vi "HEWH Create Header File.vi"(8 "Supply Voltage:":string, 9 "Test_Type:":string, 10 "HEWH Output Information":T1={"Scan Rate Adjust"=1000.0, "Draw Count"=0, "Test Patten Setup"={"Dispense Times"=[0.0, 3600.0, 7200.0, 10800.0, 14400.0, 18000.0], "Total Gallons Schedule"=[10.72, 10.72, 10.72, 10.72, 10.72, 10.72], "Flow Rate Schedule "=[3.0, 3.0, 3.0, 3.0, 3.0, 3.0], "Incoming Water Temperature"=[58.0, 58.0, 58.0, 58.0, 58.0, 58.0], "PreDraw Pattern"=[], "24 Hour PreDraw"=enum."Zero Pre-Draws", "Pre-Draw Until?"=[], "Purge Until Cutout"=FALSE, "Heating Flag"=FALSE}, "Condition Cluster Output"={"Condition #1"=FALSE, "Condition #2"=FALSE, "Special Last Draw (HU Test)"=FALSE, "RTD Out Temperature <="=0.0, "Condition #3"=FALSE, "Mean Tank Temperature <="=0.0, "Condition #4"=FALSE, "Decrease Outlet Temperature \nBy (RTD Out)"=0.0, "Condition #5"=FALSE, "Condition #6"=FALSE, "Time (Seconds)"=0.0, "Condition #7"=FALSE, "Condition #8"=FALSE, "Draw Until Condition"={"UE"=FALSE, "LE"=FALSE, "COMP"=FALSE, "FANS"=FALSE}, "Condition #9"=FALSE}, "HEWH Specific DAQ"={"HEWH Data"={"Voltage (Volts)"=-1.0, "Current (Amps)"=-1.0, "Power (Watts)"=-1.0, "WattHours (Wh)"=-1.0, "TC Tree (AVG)"=0.0, "Flow Rate (GPM)"=0.0, "Gallons (Gal)"=0.0, "RTD Out (Deg F)"=0.0, "TC Down"=0.0, "TC Tree Array"=[], "UE Event Lead"=0, "LE Event Lead"=0}, "Intellif Valve % Open"=0.0, "Power State"={"UE"=FALSE, "LE"=FALSE, "COMP"=FALSE, "FANS"=FALSE}, "Power Analyzer"=enum."APLUS", "Intellifaucet Configuration"=enum."DRK375,STATION3,1/2\"HOSE"}, "Test Output Data"={"PreDraw Data Table"=[], "Data Table"=[], "MW100 TC Headers"=[]}, "Calc and Calibration"={"RTD Max Min Array"=[], "Draw Statistics"=[], "Calibration Coefficients DBL"=[], "Min RTD Temp\nDuring Draw"=0.0, "Start Gallons"=0.0, "Starting Temp Decline Temp"=0.0, "Max RTD Temp\nDuring Draw"=0.0, "Draw Start Time"=0.0, "Delay Start Time"=0.0, "Current Purge Start Time"=0.0}, "Current Draw Time"=0.0} {"Test Patten Setup"."Incoming Water Temperature" format="%.2f"; "Test Patten Setup"."Flow Rate Schedule" format="%.2f"; "Test Patten Setup"."Total Gallons Schedule" format="%.2f"; "Test Patten Setup"."Dispense Times" format="%<%H:%M:%S>t"}) -> (3 "File Initialization Array":string[][](array[string]))   [LabVIEW 2016]
uses:
  Hybrid Water Heater/Type Definitions/HEWH Output Information.ctl
  Hybrid Water Heater/Type Definitions/HEWH Power Data.ctl
  Hybrid Water Heater/Type Definitions/HEWH Draw Pattern Setup.ctl
  Hybrid Water Heater/Type Definitions/HEWH Power Elements.ctl
  Hybrid Water Heater/Type Definitions/HEWH Termination Condition Cluster.ctl
  Hybrid Water Heater/Type Definitions/HEWH PreDraw.ctl
  Type Definitions/UTILITY Power Analyzer.ctl
  Hybrid Water Heater/Custom Instrument Control/Intellifaucet/Type Definitions/INTELLIFAUCET Tested Flowrate Scenarios.ctl
panel:
  # "Select Only One Condition"
  # "Just Draw Water!"
  # "Condition #1"
  # "Draw Until Any Heat Source"
  # "Condition #2"
  # "Start Dispense Pattern"
  # "Draw Until Specific Heat Source"
  # "Condition #3"
  # "Dispense PRAT Sequence"
  # "Not Working"
  # "Condition #4"
  # "Condition #5"
  # "Condition #6"
  # "Draw Pattern Setup"
  # "Pre-Draw Items"
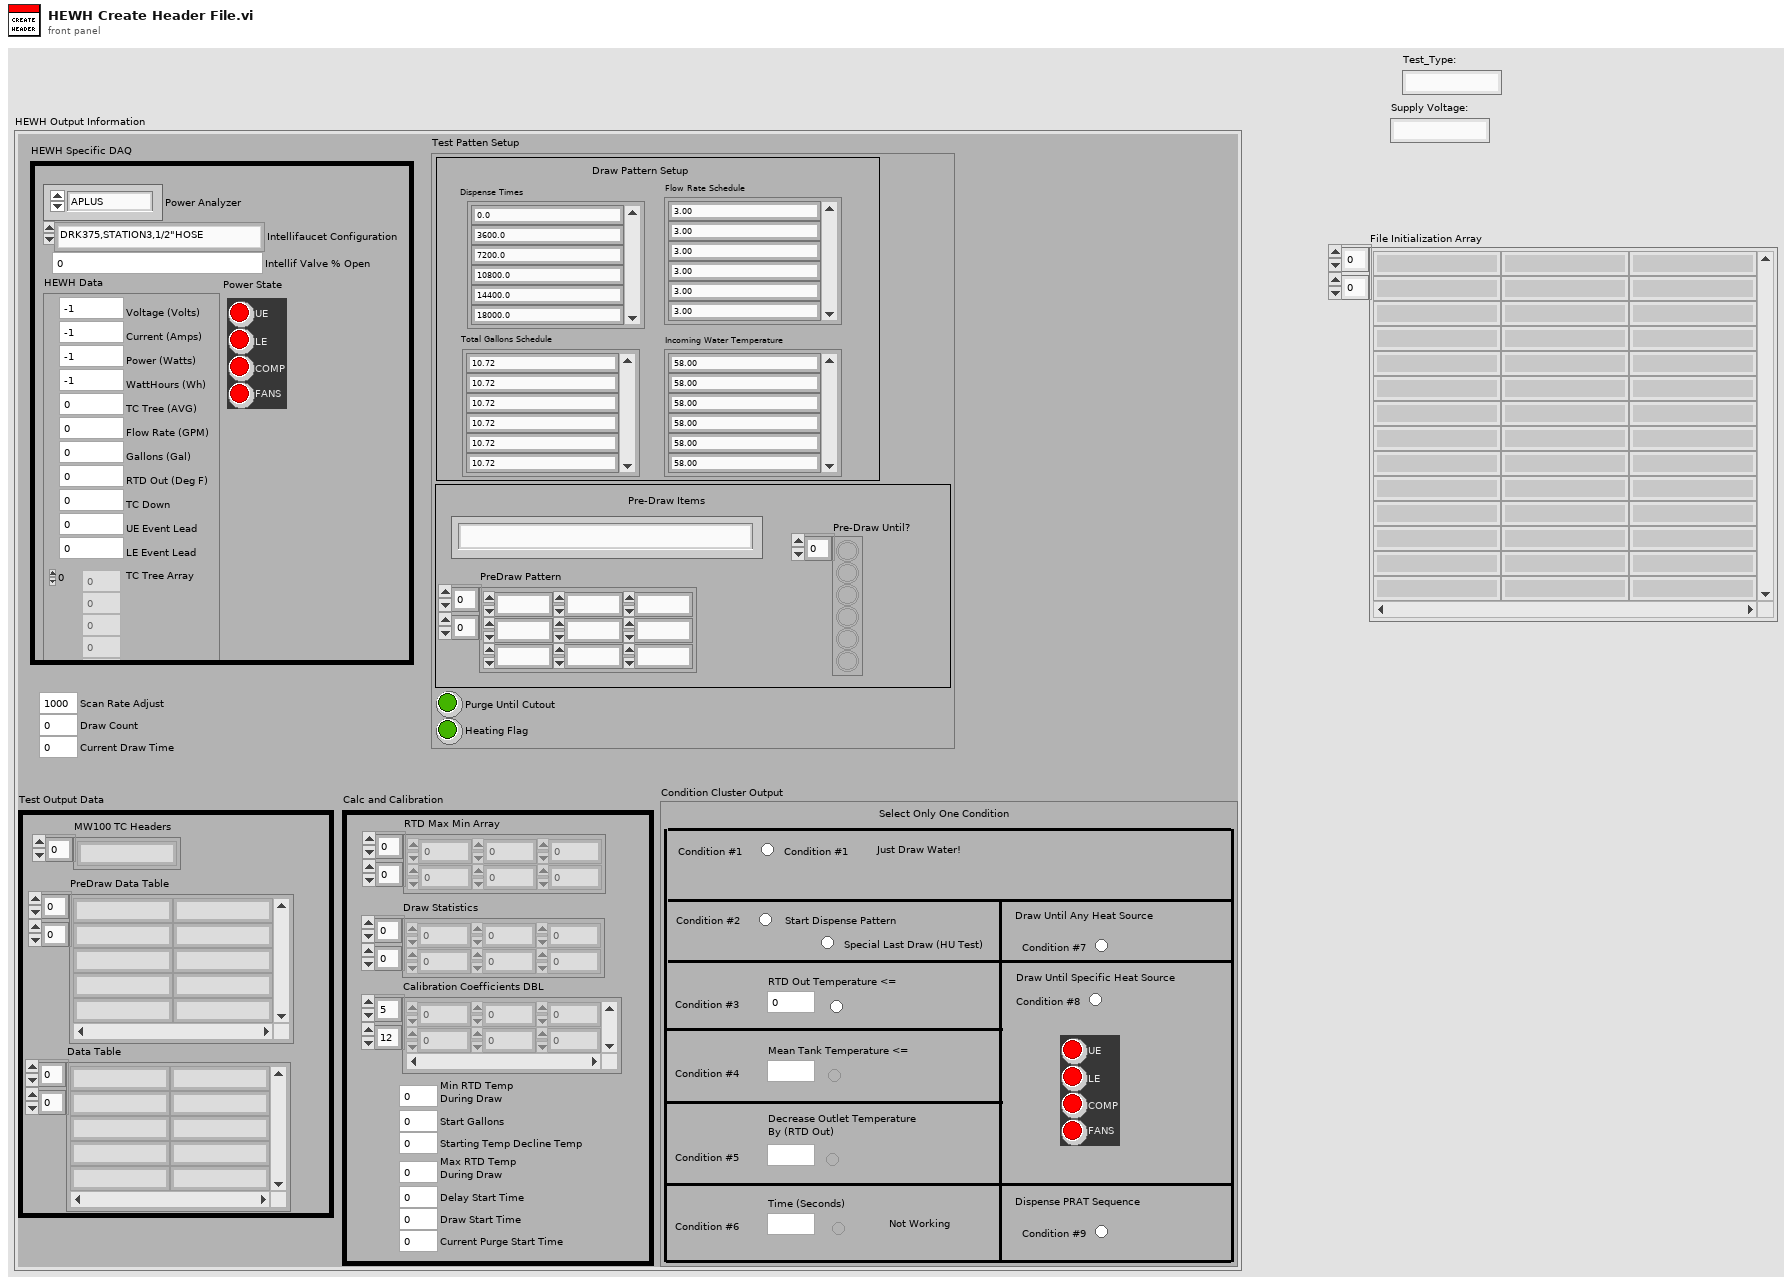
[diagram p1: front panel]
types:
  T1 = typedef "HEWH Output Information.ctl" = cluster{"Scan Rate Adjust":dbl, "Draw Count":i32, "Test Patten Setup":T2, "Condition Cluster Output":T4, "HEWH Specific DAQ":cluster{"HEWH Data":T6, "Intellif Valve % Open":dbl, "Power State":T5, "Power Analyzer":T7, "Intellifaucet Configuration":T8}, "Test Output Data":cluster{"PreDraw Data Table":string[][], "Data Table":string[][], "MW100 TC Headers":string[]}, "Calc and Calibration":cluster{"RTD Max Min Array":dbl[][], "Draw Statistics":dbl[][], "Calibration Coefficients DBL":dbl[][], "Min RTD Temp\nDuring Draw":dbl, "Start Gallons":dbl, "Starting Temp Decline Temp":dbl, "Max RTD Temp\nDuring Draw":dbl, "Draw Start Time":dbl, "Delay Start Time":dbl, "Current Purge Start Time":dbl}, "Current Draw Time":dbl}
  T2 = typedef "HEWH Draw Pattern Setup.ctl" = cluster{"Dispense Times":dbl[], "Total Gallons Schedule":dbl[], "Flow Rate Schedule ":dbl[], "Incoming Water Temperature":dbl[], "PreDraw Pattern":dbl[][], "24 Hour PreDraw":T3, "Pre-Draw Until?":bool[], "Purge Until Cutout":bool, "Heating Flag":bool}
  T3 = typedef "HEWH PreDraw.ctl" = enum16{"Zero Pre-Draws", "One Pre- Draws", "Two Pre-Draws", "Three Pre-Draws", ""}
  T4 = typedef "HEWH Termination Condition Cluster.ctl" = cluster{"Condition #1":bool, "Condition #2":bool, "Special Last Draw (HU Test)":bool, "RTD Out Temperature <=":dbl, "Condition #3":bool, "Mean Tank Temperature <=":dbl, "Condition #4":bool, "Decrease Outlet Temperature \nBy (RTD Out)":dbl, "Condition #5":bool, "Condition #6":bool, "Time (Seconds)":dbl, "Condition #7":bool, "Condition #8":bool, "Draw Until Condition":T5, "Condition #9":bool}
  T5 = typedef "HEWH Power Elements.ctl" = cluster{"UE":bool, "LE":bool, "COMP":bool, "FANS":bool}
  T6 = typedef "HEWH Power Data.ctl" = cluster{"Voltage (Volts)":dbl, "Current (Amps)":dbl, "Power (Watts)":dbl, "WattHours (Wh)":dbl, "TC Tree (AVG)":dbl, "Flow Rate (GPM)":dbl, "Gallons (Gal)":dbl, "RTD Out (Deg F)":dbl, "TC Down":dbl, "TC Tree Array":dbl[], "UE Event Lead":i32, "LE Event Lead":i32}
  T7 = typedef "UTILITY Power Analyzer.ctl" = enum16{"", "APLUS", "WT210", "WT500", "WT300", "OSI", "Debug", "WT230", "WT300_1", "WT300_2"}
  T8 = typedef "INTELLIFAUCET Tested Flowrate Scenarios.ctl" = enum16{"DRK500,Station1", "DRK375,Lab", "SRK500,Station1,5GPM FR", "DRK375,STATION3,1/2\"HOSE", "DRK500,Station1,downspout", "DRK375,Station3,thruEcocute", "DRK375,Station3,purge", "Build2,2B,Purge", "Global, Purge", "Global, Tank", "DRK250"}
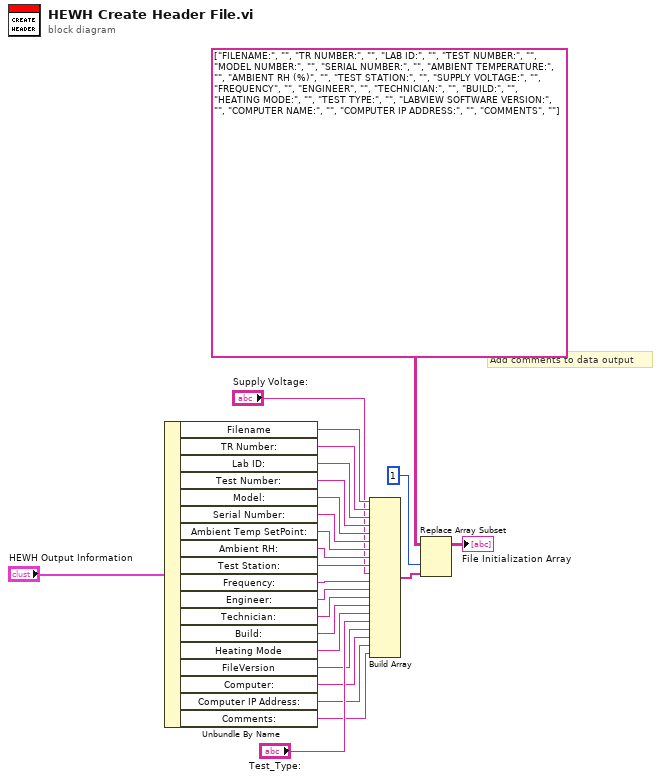
[diagram p0: block diagram]
diagram:
  # "Add comments to data output"
  n1 = Unbundle By Name("HEWH Output Information") -> ("Filename"=w21:string, "TR Number:"=w20:string, "Lab ID:"=w19:string, "Test Number:"=w18:string, "Model:"=w17:string, "Serial Number:"=w16:string, "Ambient Temp SetPoint:"=w15:string, "Ambient RH:"=w14:string, "Test Station:"=w13:string, "Frequency:"=w11:string, "Engineer:"=w10:string, "Technician:"=w9:string, "Build:"=w8:string, "Heating Mode"=w7:string, "FileVersion"=w4:string, "Computer:"=w3:string, "Computer IP Address:"=w2:string, "Comments:"=w1:string)
  n2 = Build Array(w21, w20, w19, w18, w17, w16, w15, w14, w13, "Supply Voltage:", w11, w10, w9, w8, w7, "Test_Type:", w4, w3, w2, w1) -> (w5:string[])
  n3 = Replace Array Subset(array=string[][] [["FILENAME:", ""], ["TR NUMBER:", ""], ["LAB ID:", ""], ["TEST NUMBER:", ""], ["MODEL NUMBER:", ""], ["SERIAL NUMBER:", ""], ["AMBIENT TEMPERATURE:", ""], ["AMBIENT RH (%)", ""], ["TEST STATION:", ""], ["SUPPLY VOLTAGE:", ""], ["FREQUENCY", ""], ["ENGINEER", ""], ["TECHNICIAN:", ""], ["BUILD:", ""], ["HEATING MODE:", ""], ["TEST TYPE:", ""], ["LABVIEW SOFTWARE VERSION:", ""], ["COMPUTER NAME:", ""], ["COMPUTER IP ADDRESS:", ""], ["COMMENTS", ""]], new element=w5, index (col)=1 ("disabled index (col)")) -> (→"File Initialization Array":string[][])  [unwired: 1 in]
